vi "Sweep Control.vi"(1 "Stop":bool, 4 "Experiment Description":string="IV measurements at 0T\n- Sweep priority 0: +x gate from -10V to 10V in steps of 500mV (-x 10 to -10)\n- priority 1:+y gate from -10V to 10V in steps of 500mV (-y 10 to -10)\n- 1 IV curves at each Vsg\n- KH channel 17,18,19,20: leads 3,8,15,21\n- 5 s wait\n\nVbg = lead 26: 0V\nT: 20mK\nB=0T\n\nhash device\n\nKH channel 10,13: leads 16,27 , current mode, 5k resistor, 1000x gain\nlead 16: 3mV ac+ 1mV dc bias, 1 Hz\nKH channel 11,12: V1+/-: 17/20, 100x gain\nKH channel 5: dV: 17-20, 100x gain\n\nstripe device\n\nKH channel 7,8: leads 11,12 , current mode, 5k resistor, 1000x gain\nlead 12: 3.5mV ac+ 0mV dc bias, 1 Hz\nKH channel 6,9: V1+/-: 9,13, 100x gain\nKH channel 16: dV: 11-12, 100x gain", 5 "Experiment subVI":T9, 6 "Sweep Lockin":T1[](array[typedef]) {"Channels"."Table" format="%#_1f"; "Channels"."Channel" min=1 max=128; "Channels"."Start" format="%#_6p"; "Channels"."End" format="%#_6p"}, 7 "Experiment Folder (## - Description)":string="35-2D_0T_IV_hash_stripe", 8 "error in (no error)":errorcluster, 9 "Post action (indexing priority)":T10=[enum."Do Nothing", enum."Do Nothing", enum."Do Nothing", enum."Do Nothing"], 10 "Scan parameters":T12=[{"Start"=0.0, "End"=0.0, "Step"=0.0, "Rate"=0.0, "Waveform type"=enum."linear", "wait (ms or K)"=0.0, "Address"="Dev2/ao0", "channel"=17}, {"Start"=0.0, "End"=0.0, "Step"=0.0, "Rate"=0.0, "Waveform type"=enum."linear", "wait (ms or K)"=0.0, "Address"="Dev2/ao0", "channel"=18}, {"Start"=0.0, "End"=0.0, "Step"=0.0, "Rate"=0.0, "Waveform type"=enum."linear", "wait (ms or K)"=0.0, "Address"="Dev2/ao0", "channel"=19}, {"Start"=0.0, "End"=0.0, "Step"=0.0, "Rate"=0.0, "Waveform type"=enum."linear", "wait (ms or K)"=0.0, "Address"="Dev2/ao0", "channel"=20}] {"Rate" format="%.2f"; "Step" format="%#_6p"; "End" format="%#_6p"; "Start" format="%#_6p"}, 11 "Scan control":T14=[{"Priority"=enum."Priority 0", "Scan name"=enum."Lockin Bias"}, {"Priority"=enum."Priority 1", "Scan name"=enum."Lockin Bias"}, {"Priority"=enum."Priority 0", "Scan name"=enum."Lockin Bias"}, {"Priority"=enum."Priority 1", "Scan name"=enum."Lockin Bias"}]) -> (0 "error out":errorcluster)   [LabVIEW 2019, in "SMO.SweepControl.lvclass"]
doc: "- Priority 0 is the fastest loop\n- You can put multiple scan names in one priority.\n- OFF has to be the last priority\n- Choose an Experiment (Lockin_Sweep, IV, etc) to run at each Scan Setting\n- Open the Exeriment subVIs to choose settings"
uses:
  SMO.SweepControl.lvclass
  Typedefs/Enum - Priority.ctl
  Typedefs/Enum - Action.ctl
  Typedefs/Cluster - ScanControl.ctl
  Typedefs/ScanControl.ctl
  Typedefs/Cluster - ScanParamters.ctl
  Typedefs/ScanParamters.ctl
  Typedefs/Enum - Experiments.ctl
  Typedefs/Sweep Control JSON--Cluster.ctl
  SMO.Control Experiment/SMO.Control Experiment.lvclass
  Control Experiment SM/Control Experiment SM.lvclass
  Typedefs/Enum - PostAction.ctl
  Typedefs/PostAction.ctl
  Typedefs/Enum - PostAction - 2.ctl
  Typedefs/Cluster - Sweep Control.ctl
  <userlib>/LevyLab/Lockin-Multichannel/Instrument.DAQ/Typedefs/Sweep.Pattern--Enum.ctl
  <userlib>/LevyLab/Lockin-Multichannel/Instrument.DAQ/Instrument.DAQ.lvclass
  <userlib>/LevyLab/Lockin-Multichannel/Instrument.DAQ/Typedefs/Sweep.Channel--Cluster.ctl
  <userlib>/LevyLab/Lockin-Multichannel/Instrument.DAQ/Typedefs/Sweep.Channel--Cluster--Array.ctl
  <userlib>/LevyLab/Lockin-Multichannel/Instrument.DAQ/Typedefs/Sweep.Configuration--Cluster.ctl
panel:
  out "Repeat #":i32
  in  "Repeat Experiment":i32=1 caption="Repeat Experiment (at each parameter)" min=1
  in  "Scan parameters 2":T5[](array[typedef]) {"Rate" format="%.2f"; "Step" format="%#_6p"; "End" format="%#_6p"; "Start" format="%#_6p"}
  # "1. Scan Parameters. Choose parameters at which each experiment will take place."
  # "2. Experiment"
  # "3. If your chosen experiment is \"Lockin Sweep\", then the following sequence of sweeps will be executed at each scan parameter. (Ex. 1. Set B. 2. Set Set Vsg. 3. Lockin Sweep 1. 4. Lockin Sweep 2. Etc."
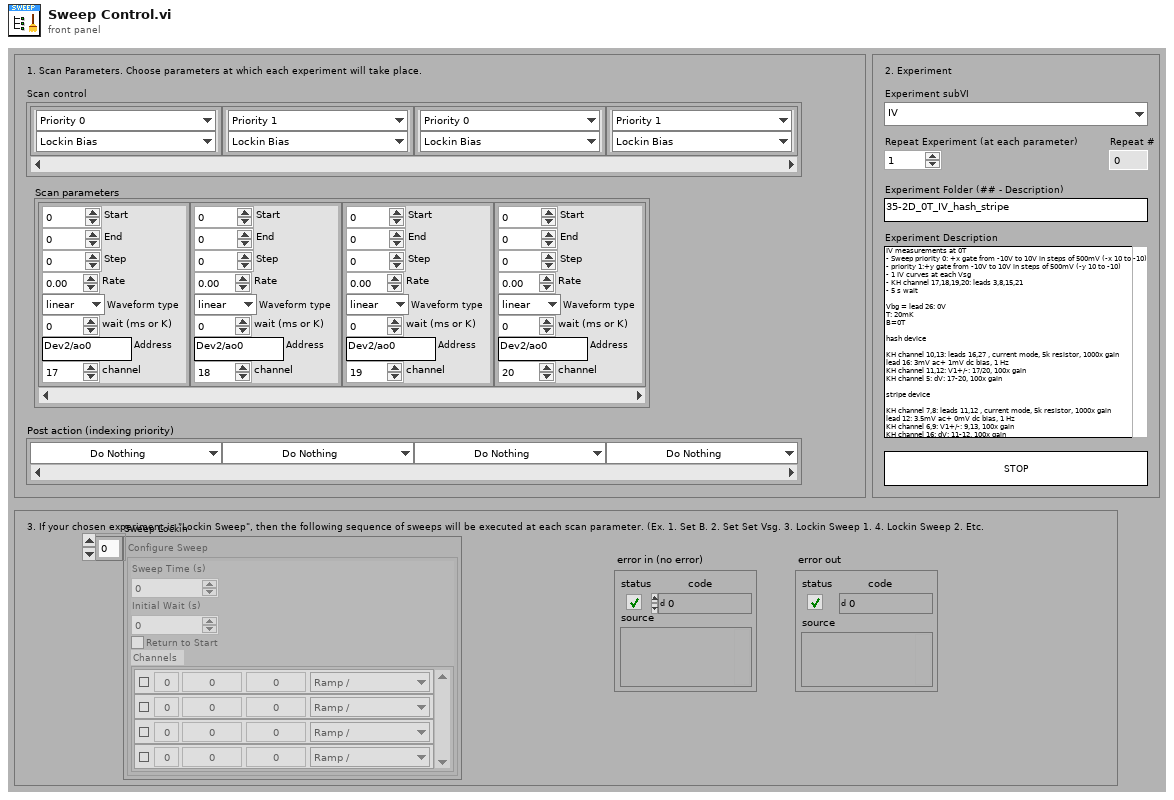
[diagram p1: front panel]
types:
  T1 = typedef "Instrument.DAQ.lvclass/Sweep.Configuration--Cluster.ctl" = cluster{"Sweep Time (s)":dbl, "Initial Wait (s)":dbl, "Return to Start":bool, "Channels":T2}
  T2 = typedef "Instrument.DAQ.lvclass/Sweep.Channel--Cluster--Array.ctl" = T3[]
  T3 = typedef "Instrument.DAQ.lvclass/Sweep.Channel--Cluster.ctl" = cluster{"Enable?":bool, "Channel":u16, "Start":dbl, "End":dbl, "Pattern":T4, "Table":dbl[]}
  T4 = typedef "Instrument.DAQ.lvclass/Sweep.Pattern--Enum.ctl" = enum16{"Ramp /", "Ramp /\\", "Smooth Ramp _/", "Smooth Ramp _/\\_", "Table"}
  T5 = typedef "SMO.SweepControl.lvclass/Cluster - Sweep Control.ctl" = cluster{"Start":dbl, "End":dbl, "Step":dbl, "Rate":dbl, "wait (ms/mK)":u32, "Address":string, "Priority":T6, "Scan name":T7, "Post Actions":T8[], "channel":i32}
  T6 = typedef "SMO.SweepControl.lvclass/Enum - Priority.ctl" = enum16{"Priority 0", "Priority 1", "Priority 2", "Priority 3", "Priority 4", "Priority 5"}
  T7 = typedef "SMO.SweepControl.lvclass/Enum - Action.ctl" = enum16{"OFF", "time", "Lockin Amplitude", "Lockin Frequency", "Lockin Bias", "Delay", "Strain", "DAQ Bias", "Magnet Field", "Temperature", "MW f1", "MW f2", "MW Amplitude1", "MW Amplitude2"}
  T8 = typedef "SMO.SweepControl.lvclass/Enum - PostAction - 2.ctl" = enum16{"Do Nothing", "Wait (time)", "Wait (Temperature)", "Wait (<T ; B sweep)", "Wait (Magnet)"}
  T9 = typedef "SMO.SweepControl.lvclass/Enum - Experiments.ctl" = enum16{"IV", "IV_Fast", "THz_DelayLine", "Lockin_Vsg", "Lockin_Sweep", "Lockin_Time", "AI WFM time", "Lockin (experimental)"}
  T10 = typedef "SMO.SweepControl.lvclass/PostAction.ctl" = T11[]
  T11 = typedef "SMO.SweepControl.lvclass/Enum - PostAction.ctl" = enum16{"Do Nothing", "Wait (time)", "Wait (Temperature)", "Wait (<T ; B sweep)", "Wait (Magnet)"}
  T12 = typedef "SMO.SweepControl.lvclass/ScanParamters.ctl" = T13[]
  T13 = typedef "SMO.SweepControl.lvclass/Cluster - ScanParamters.ctl" = cluster{"Start":dbl, "End":dbl, "Step":dbl, "Rate":dbl, "Waveform type":enum16{"linear", "triangle", "power"}, "wait (ms or K)":dbl, "Address":string, "channel":i32}
  T14 = typedef "SMO.SweepControl.lvclass/ScanControl.ctl" = T15[]
  T15 = typedef "SMO.SweepControl.lvclass/Cluster - ScanControl.ctl" = cluster{"Priority":T6, "Scan name":T7}
  T16 = enum32{"Invalid", "Standard", "Closed", "Hidden", "Minimized", "Maximized"}
  T17 = enum32{"invalid app kind", "Development System", "Run Time System", "Student Edition", "Embedded LabVIEW", "Evaluation", "Custom"}
  T18 = cluster{"Core":cluster{"Current VI Reference":refnum<vi>, "Close Panel on Exit?":bool}, "SweepControl":refnum<class "SMO.SweepControl.lvclass">}
  T19 = cluster{"Current VI Reference":refnum<vi>, "Close Panel on Exit?":bool}
  T20 = typedef "SMO.SweepControl.lvclass/Sweep Control JSON--Cluster.ctl" = cluster{"Experiment":T9, "Repeat Experiment":i32, "Scan control":T14, "Scan parameters":T12}
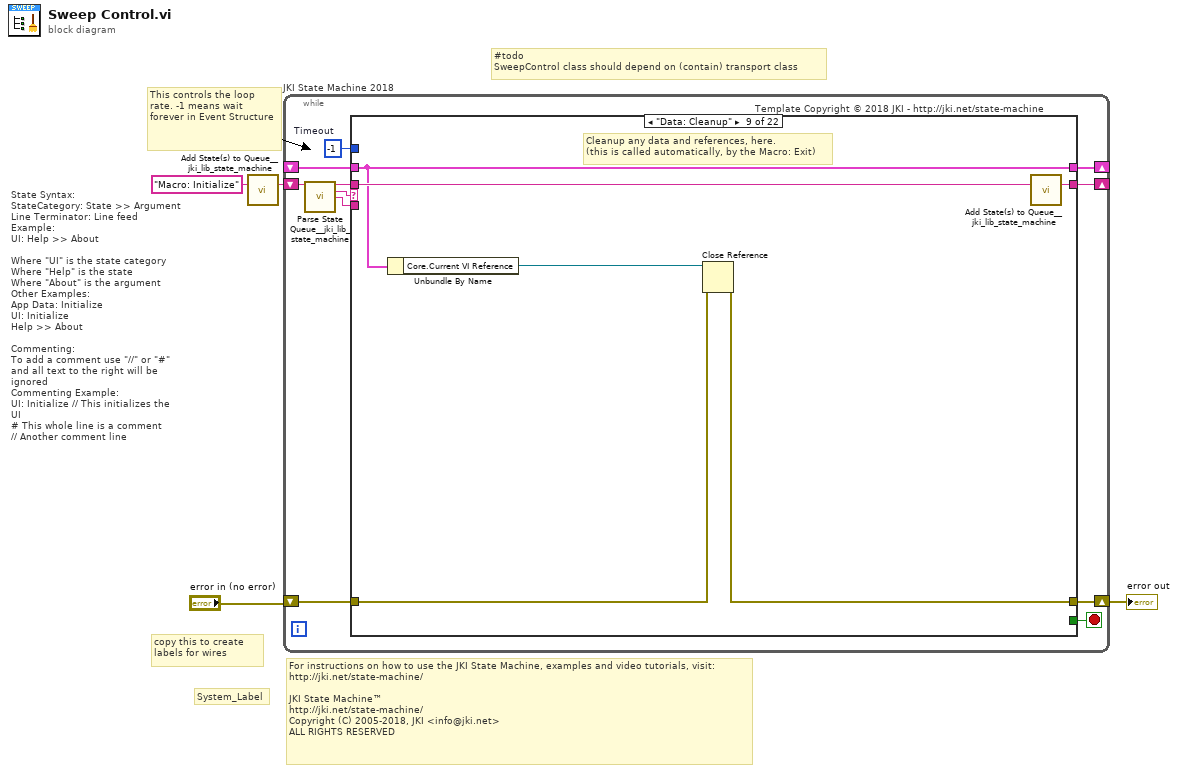
[diagram p0: block diagram]
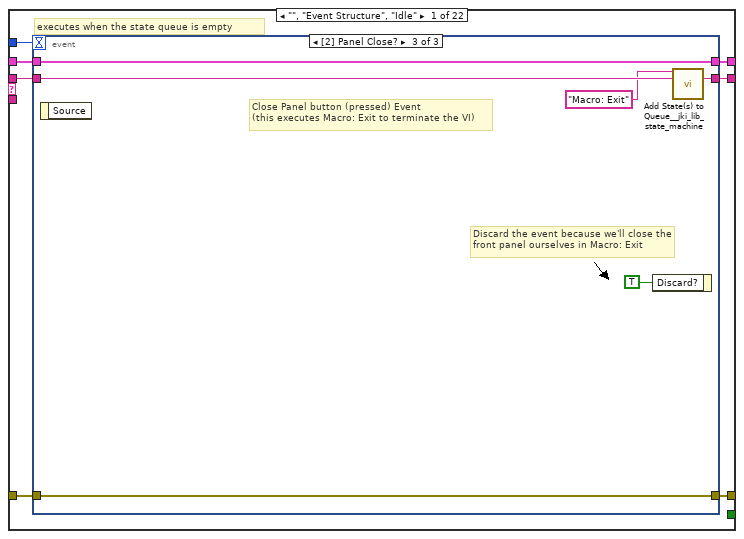
[diagram p2: hidden frame]
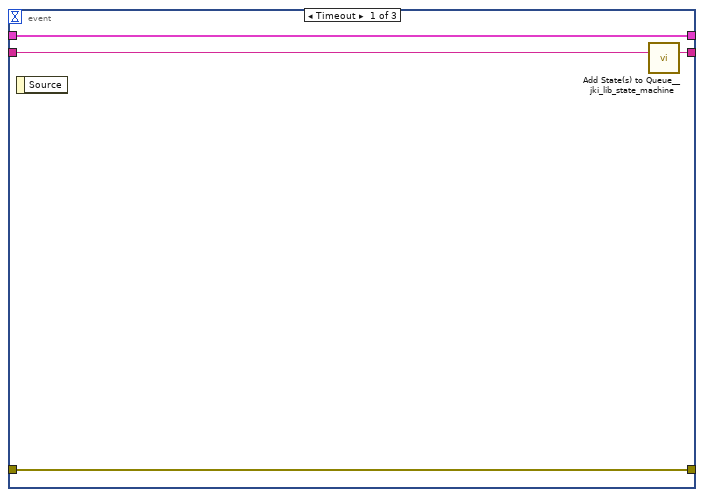
[diagram p3: hidden frame]
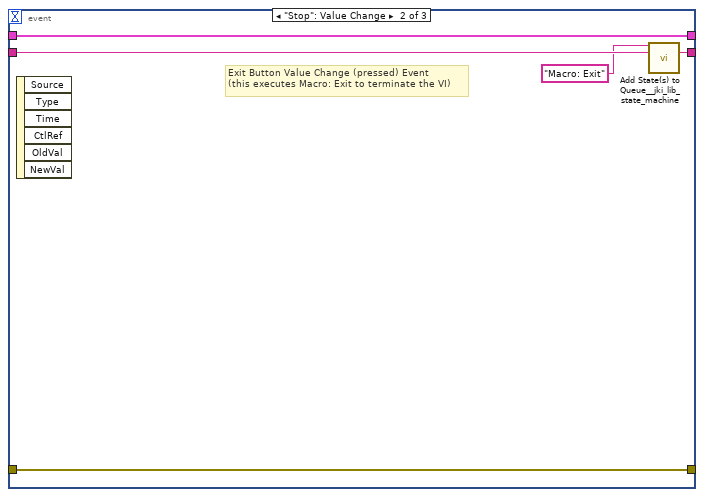
[diagram p4: hidden frame]
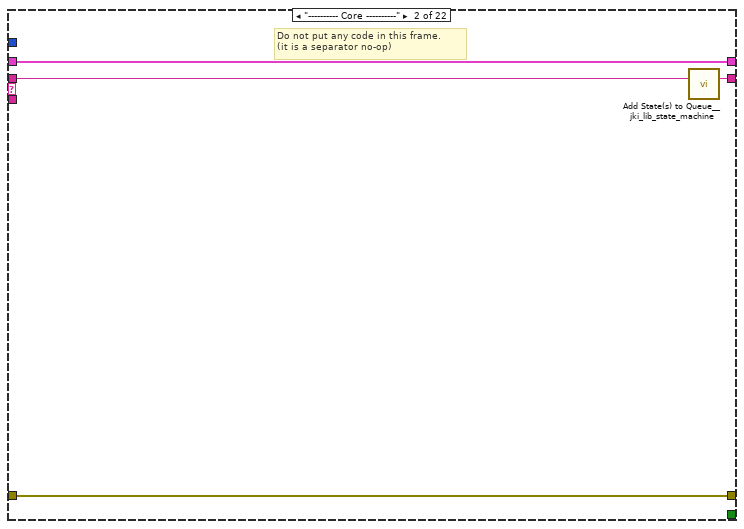
[diagram p5: hidden frame]
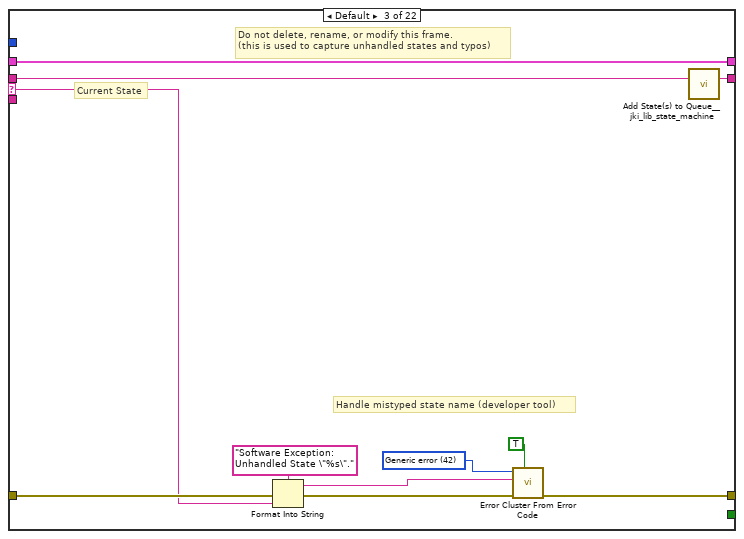
[diagram p6: hidden frame]
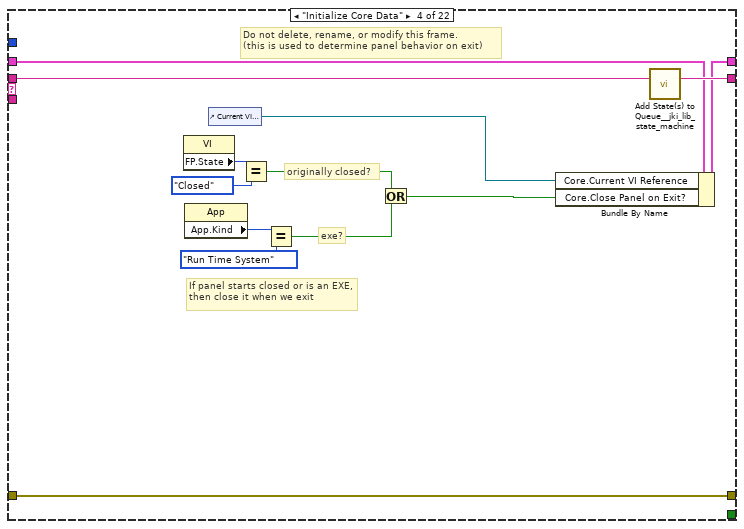
[diagram p7: hidden frame]
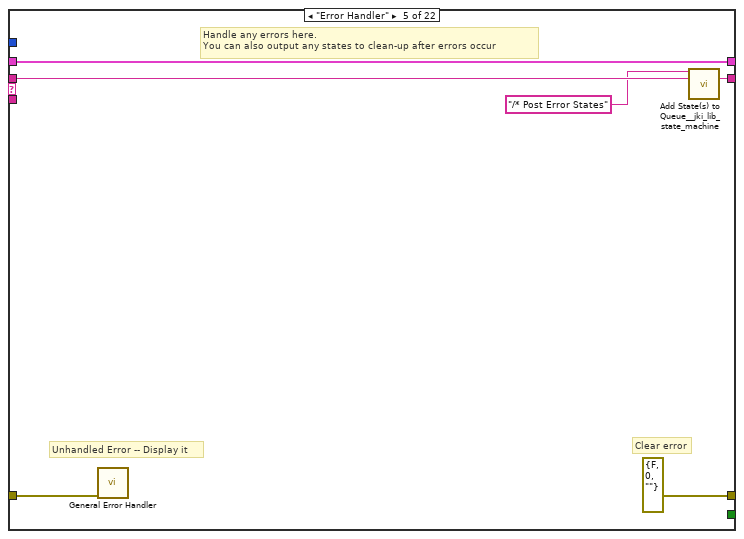
[diagram p8: hidden frame]
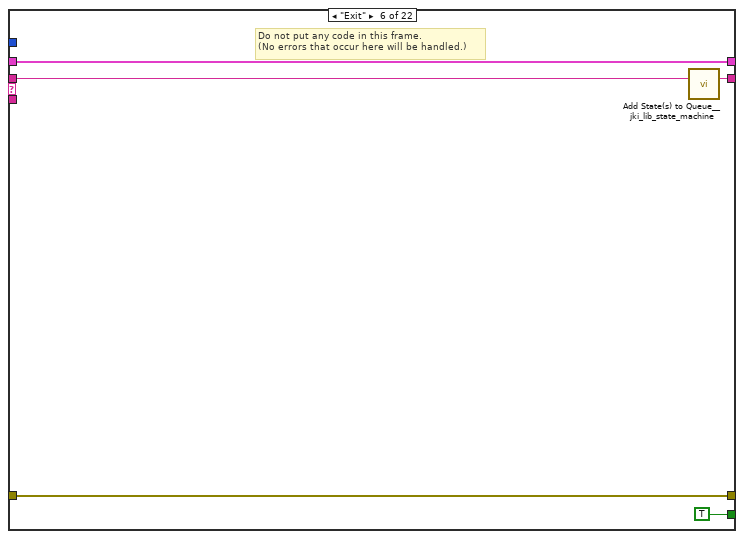
[diagram p9: hidden frame]
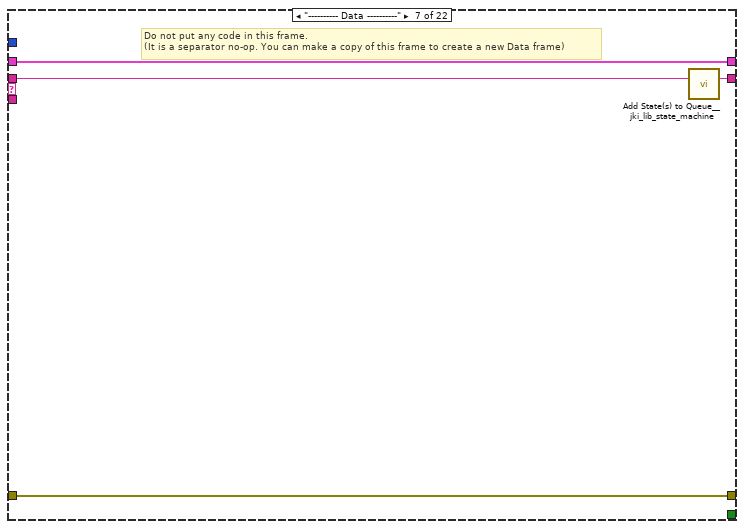
[diagram p10: hidden frame]
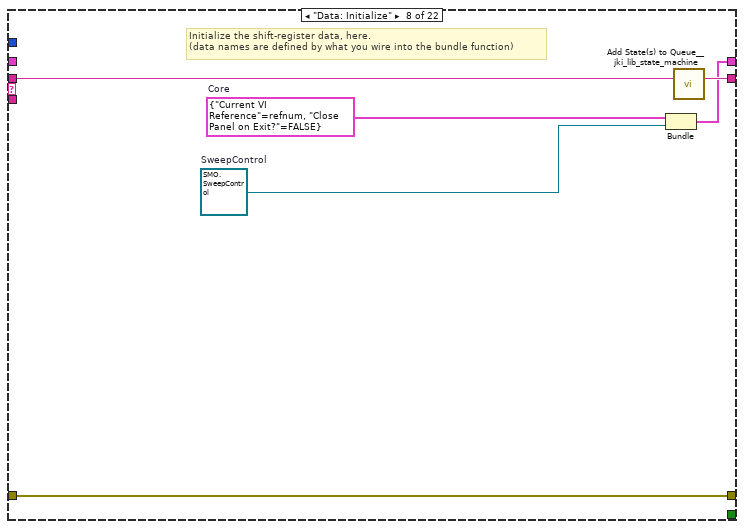
[diagram p11: hidden frame]
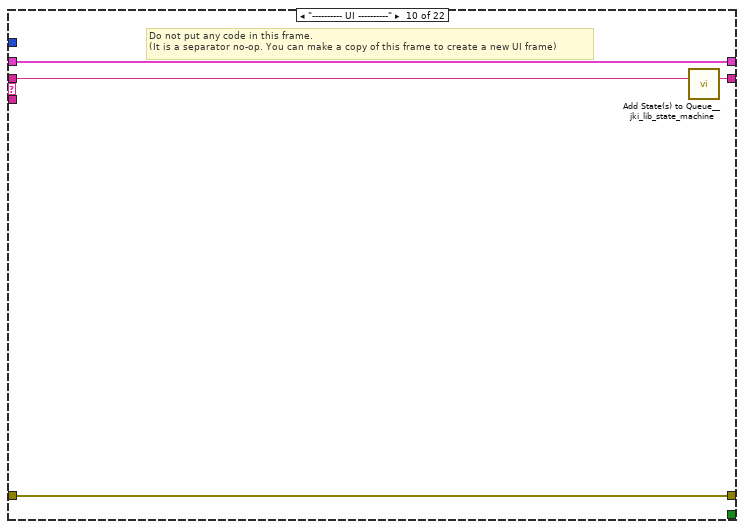
[diagram p12: hidden frame]
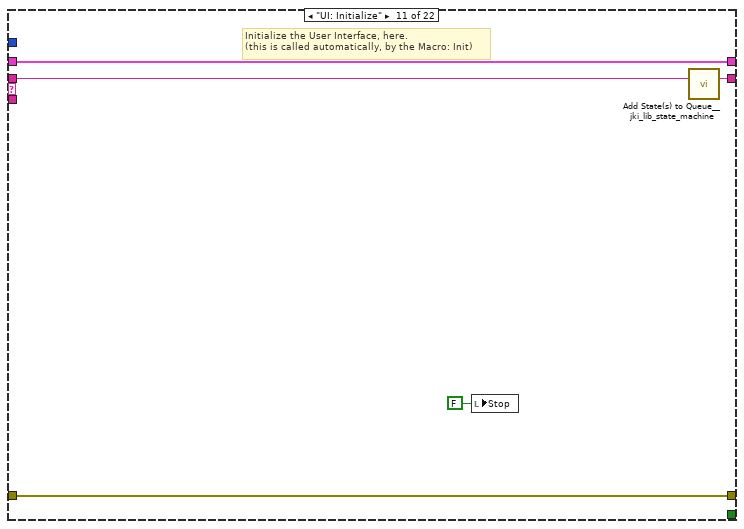
[diagram p13: hidden frame]
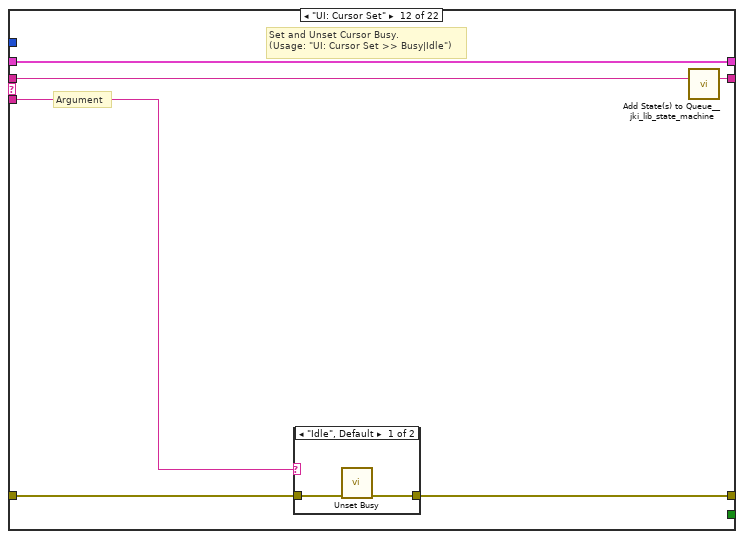
[diagram p14: hidden frame]
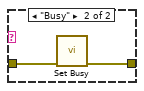
[diagram p15: hidden frame]
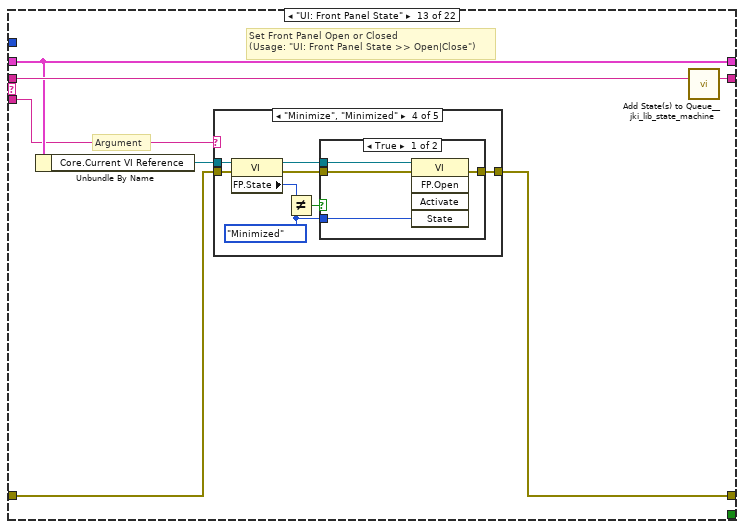
[diagram p16: hidden frame]
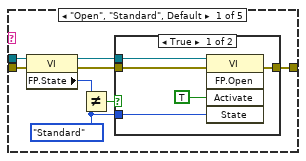
[diagram p17: hidden frame]
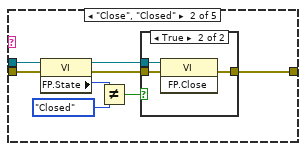
[diagram p19: hidden frame]
diagram:
  # "For instructions on how to use the JKI State Machine, examples and video tutorials, visit:\nhttp://jki.net/state-machine/\n\nJKI State Machine™\nhttp://jki.net/state-machine/\nCopyright (C) 2005-2018, JKI <info@jki.net>\nALL RIGHTS RESERVED"
  # "State Syntax:\nStateCategory: State >> Argument\nLine Terminator: Line feed\nExample:\nUI: Help >> About\n\nWhere \"UI\" is the state category\nWhere \"Help\" is the state\nWhere \"About\" is the argument\nOther Examples:\nApp Data: Initialize\nUI: Initialize\nHelp >> About\n\nCommenting:\nTo add a comment use \"//\" or \"#\" and all text to the right will be ignored\nCommenting Example:\nUI: Initialize // This initializes the UI\n# This whole line is a comment\n// Another comment line"
  # "copy this to create labels for wires"
  # "This controls the loop rate. -1 means wait forever in Event Structure"
  # "System_Label"
  # "#todo\nSweepControl class should depend on (contain) transport class"
  n1 = call <vilib>:"Add State(s) to Queue__jki_lib_state_machine.vi"("State(s) in (\"\")"="Macro: Initialize") -> ("States Out"=w4:string)  [unwired: 14 in]
  n2 = while "JKI State Machine 2018" {
    shift-right: [w8] -> _
    shift-left: _ -> [w7]
    shift-right: [w11] -> w1
    shift-left: "error in (no error)" -> [w5]
    shift-right: [w10] -> _
    shift-left: w4 -> [w12]
    stop <- w9 stop-if-true
    w6 = -1  # Timeout
    # "Template Copyright © 2018 JKI - http://jki.net/state-machine"
    n3 = call <vilib>:"Parse State Queue__jki_lib_state_machine.vi"("State Queue"=w12) -> ("Remaining States"=w14:string, "Current State"=w15:string, "Arguments"=w13:string)  [unwired: 12 in]
    n4 = case shown="\"Data: Cleanup\"" w15 {
      selector: w15 -> [_ _ w42 _ _ _ _ _ _ _ _ _ _ _ _ _ _ _ _ _ _ _]
      tunnel: w14 -> [w22 w41 w46 w65 w71 w76 w80 w86 w92 w96 w101 w107 w118 w187 w192 w197 w208 w212 w238 w251 w256 w264]
      tunnel: w13 -> [_ _ _ _ _ _ _ _ _ _ _ w102 w112 _ _ _ _ _ _ _ _ _]
      tunnel: w7 -> [w20 w38 w44 w58 w68 w74 w77 _ w87 w93 w99 w105 w114 w184 w189 w194 w205 w209 w232 w249 w254 w260]
      tunnel: [w19 w39 w48 w62 errorcluster {"status"=FALSE, "code"=0, "source"=""} ("error out") w73 w78 w83 w88 w94 w98 w103 w115 w185 w190 w195 w206 w210 w230 w247 w252 w263] -> w11
      tunnel: w5 -> [w18 w39 w47 w62 w67 w73 w78 w83 w89 w94 w98 w104 w116 w185 w190 w195 w206 w210 w226 w239 w252 w263]
      tunnel: [w21 w40 w45 w64 w70 w75 w79 w85 w91 w95 w100 w106 w117 w186 w191 w196 w207 w211 w237 w250 w255 w265] -> w10
      tunnel: [_ _ _ _ _ TRUE _ _ _ _ _ _ _ _ _ _ _ _ _ _ _ _] -> w9
      tunnel: [w17 w38 w44 w63 w68 w74 w77 w84 w87 w93 w99 w105 w114 w184 w189 w194 w205 w209 w231 w249 w254 w259] -> w8
      tunnel: w6 -> [w16 _ _ _ _ _ _ _ _ _ _ _ _ _ _ _ _ _ _ _ _ _]
      frame "", "Event Structure", "Idle" {
        # "executes when the state queue is empty"
        n5 = event shown="[2] Panel Close?" {
          selector: _ -> [_ _ _]
          dyn-events: _ -> [_ _ _]
          timeout: w16 -> [_ _ _]
          tunnel: w22 -> [w26 w31 w37]
          tunnel: [w25 w30 w36] -> w21
          tunnel: w20 -> [w23 w28 w34]
          tunnel: [w24 w29 w35] -> w19
          tunnel: w18 -> [w24 w29 w35]
          tunnel: [w23 w28 w34] -> w17
          event Timeout {
            n6 = event-data() -> ()  [unwired: 1 in, 1 out]
            n7 = call <vilib>:"Add State(s) to Queue__jki_lib_state_machine.vi"("State(s) in (\"\")"=w26) -> ("States Out"=w25:string)  [unwired: 14 in]
          }
          event "Stop": Value Change {
            # "Exit Button Value Change (pressed) Event\n(this executes Macro: Exit to terminate the VI)"
            n8 = event-data() -> ()  [unwired: 1 in, 6 out]
            n9 = call <vilib>:"Add State(s) to Queue__jki_lib_state_machine.vi"("State(s) in Front (\"\")"="Macro: Exit", "State(s) in (\"\")"=w31) -> ("States Out"=w30:string)  [unwired: 13 in]
          }
          event Panel Close? {
            # "Discard the event because we'll close the front panel ourselves in Macro: Exit"
            # "Close Panel button (pressed) Event\n(this executes Macro: Exit to terminate the VI)"
            n10 = event-data() -> ()  [unwired: 1 in, 1 out]
            n11 = event-data("Discard?"=TRUE) -> ()  [unwired: 1 in, 1 out]
            n12 = call <vilib>:"Add State(s) to Queue__jki_lib_state_machine.vi"("State(s) in Front (\"\")"="Macro: Exit", "State(s) in (\"\")"=w37) -> ("States Out"=w36:string)  [unwired: 13 in]
          }
        }
      }
      frame "---------- Core ----------" {
        # "Do not put any code in this frame.\n(it is a separator no-op)"
        n13 = call <vilib>:"Add State(s) to Queue__jki_lib_state_machine.vi"("State(s) in (\"\")"=w41) -> ("States Out"=w40:string)  [unwired: 14 in]
      }
      frame Default {
        w51 = 42 items=["No error", "Argument error", "Memory is full", "Out of zone", "End of file", "File already open", "Generic file I/O error", "File not found", "File permission error", "Disk is full", "Duplicate path", "Too many files open", "System feature not enabled", "Resource file not found", "Cannot add resource", "Resource not found", "Image not found", "Image memory error", "Pen does not exist", "Config type invalid", "Config token not found", "Config parse error", "Config memory error", "Bad external code format", "Bad external code offset", "External code not present", "Null window", "Destroy window error", "Null menu", "Print aborted", "Bad print record", "Print driver error", "Windows error during printing", "Memory error during printing", "Print dialog error", "Generic print error", "Invalid device refnum", "Device not found", "Device parameter error", "Device unit error", "Cannot open device", "Device call aborted", "Generic error", "Cancelled by user", "Object ID too low", "Object ID too high", "Object not in heap", "Unknown heap", "Unknown object (invalid DefProc)", "Unknown object (DefProc not in table)", "Message out of range", "Invalid (null) method", "Unknown message", "Manager call not supported", "Bad address", "Network operation in progress", "Network operation timed out", "Connection is busy", "Network attribute not supported", "Network error", "Address in use", "System out of memory", "Connection aborted", "Connection refused", "Not connected", "Already connected", "Connection closed", "Initialization error (interapplication manager)", "Bad occurrence", "Wait on unbound occurrence handler", "Occurrence queue overflow", "Datalog type conflict", "Unused", "Unrecognized type (interapplication manager)", "Memory corrupt", "Failed to make temporary DLL", "Old CIN version", "Drag socket not found", "Failed to load drop-object", "Failed to register OLE object", "Failed to release OLE object", "Format specifier type mismatch", "Unknown format specifier", "Too few format specifiers", "Too many format specifiers", "Scan failed", "Newer CIN version", "Error converting to variant", "Runtime menu error", "Password tampered", "Variant attribute not found", "Incompatible variant data type", "Event data is not available", "Event Store is not present", "Occurrence is not found", "Event Queue is not created", "Event info is not available", "Refnum passed is NULL", "Error retrieving Class GUID", "Error retrieving CoClass GUID", "Error retrieving TypeLib GUID.", "Bad built application magic bytes.", "Specific driver is different from the specific driver associated with the Logical Name.", "There is no session opened to the class driver.", "Max Error", "MAX - Error with config objects", "MAX - Error loading configuration", "MAX - Group not supported"]
        # "Current State"
        # "Do not delete, rename, or modify this frame.\n(this is used to capture unhandled states and typos)"
        # "Handle mistyped state name (developer tool)"
        n14 = Format Into String(format string="Software Exception: Unhandled State \"%s\"." ("message"), error in=w47, w42) -> (resulting string=w50:string, error out=w49:errorcluster)  [unwired: 1 in]
        n15 = call <vilib>:"Error Cluster From Error Code.vi"("show call chain? (False)"=TRUE, "error in (no error)"=w49, "error message (\"\")"=w50, "error code (0)"=w51) -> ("error out"=w48:errorcluster)  [unwired: 5 in]
        n16 = call <vilib>:"Add State(s) to Queue__jki_lib_state_machine.vi"("State(s) in (\"\")"=w46) -> ("States Out"=w45:string)  [unwired: 14 in]
      }
      frame "Initialize Core Data" {
        # "Do not delete, rename, or modify this frame.\n(this is used to determine panel behavior on exit)"
        # "originally closed?"
        # "exe?"
        # "If panel starts closed or is an EXE, then close it when we exit"
        n17 = property class="VI"() -> ("FP.State"=w55:T16)  [unwired: 2 in, 2 out]
        n18 = property class="App"() -> ("App.Kind"=w61:T17)  [unwired: 2 in, 2 out]
        n19 = control-ref of="Current VI Reference"() -> (w56:refnum<vi>)
        n20 = Equal?(x=w55, y=T16."Closed" ("Front Panel Window:State")) -> (x = y?=w53:bool)
        n21 = Equal?(x=w61, y=T17."Run Time System" ("Application:Kind")) -> (x = y?=w59:bool)
        n22 = Or(x=w53, y=w59) -> (x .or. y?=w57:bool)
        n23 = Bundle By Name(cluster=w58, "Core.Current VI Reference"=w56, "Core.Close Panel on Exit?"=w57) -> (w63:T18)
        n24 = call <vilib>:"Add State(s) to Queue__jki_lib_state_machine.vi"("State(s) in (\"\")"=w65) -> ("States Out"=w64:string)  [unwired: 14 in]
      }
      frame "Error Handler" {
        # "Unhandled Error -- Display it"
        # "Handle any errors here.\nYou can also output any states to clean-up after errors occur"
        # "Clear error"
        n25 = call <vilib>:"General Error Handler.vi"("error in (no error)"=w67) -> ()  [unwired: 10 in, 5 out]
        n26 = call <vilib>:"Add State(s) to Queue__jki_lib_state_machine.vi"("State(s) in Front (\"\")"="/* Post Error States", "State(s) in (\"\")"=w71) -> ("States Out"=w70:string)  [unwired: 13 in]
      }
      frame "Exit" {
        # "Do not put any code in this frame.\n(No errors that occur here will be handled.)"
        n27 = call <vilib>:"Add State(s) to Queue__jki_lib_state_machine.vi"("State(s) in (\"\")"=w76) -> ("States Out"=w75:string)  [unwired: 14 in]
      }
      frame "---------- Data ----------" {
        # "Do not put any code in this frame.\n(It is a separator no-op. You can make a copy of this frame to create a new Data frame)"
        n28 = call <vilib>:"Add State(s) to Queue__jki_lib_state_machine.vi"("State(s) in (\"\")"=w80) -> ("States Out"=w79:string)  [unwired: 14 in]
      }
      frame "Data: Initialize" {
        w81 = refnum<class "SMO.SweepControl.lvclass"> refnum  # SweepControl
        w82 = T19 {"Current VI Reference"=refnum, "Close Panel on Exit?"=FALSE}  # Core
        # "Initialize the shift-register data, here.\n(data names are defined by what you wire into the bundle function)"
        n29 = Bundle("Core"=w82, "SweepControl"=w81) -> (w84:T18)  [unwired: 1 in]
        n30 = call <vilib>:"Add State(s) to Queue__jki_lib_state_machine.vi"("State(s) in (\"\")"=w86) -> ("States Out"=w85:string)  [unwired: 14 in]
      }
      frame "Data: Cleanup" {
        # "Cleanup any data and references, here.\n(this is called automatically, by the Macro: Exit)"
        n31 = Unbundle By Name(w87) -> ("Core.Current VI Reference"=w90:refnum<vi>)
        n32 = Close Reference(reference=w90, error in (no error)=w89) -> (error out=w88:errorcluster)
        n33 = call <vilib>:"Add State(s) to Queue__jki_lib_state_machine.vi"("State(s) in (\"\")"=w92) -> ("States Out"=w91:string)  [unwired: 14 in]
      }
      frame "---------- UI ----------" {
        # "Do not put any code in this frame.\n(It is a separator no-op. You can make a copy of this frame to create a new UI frame)"
        n34 = call <vilib>:"Add State(s) to Queue__jki_lib_state_machine.vi"("State(s) in (\"\")"=w96) -> ("States Out"=w95:string)  [unwired: 14 in]
      }
      frame "UI: Initialize" {
        # "Initialize the User Interface, here.\n(this is called automatically, by the Macro: Init)"
        n35 = local write "Stop"(FALSE ("Stop")) -> ()
        n36 = call <vilib>:"Add State(s) to Queue__jki_lib_state_machine.vi"("State(s) in (\"\")"=w101) -> ("States Out"=w100:string)  [unwired: 14 in]
      }
      frame "UI: Cursor Set" {
        # "Argument"
        # "Set and Unset Cursor Busy.\n(Usage: \"UI: Cursor Set >> Busy|Idle\")"
        n37 = case shown="\"Idle\", Default" w102 {
          tunnel: w104 -> [w109 w111]
          tunnel: [w108 w110] -> w103
          frame "Idle", Default {
            n38 = call <vilib>:"Unset Busy.vi"("error in (no error)"=w109) -> ("error out"=w108:errorcluster)  [unwired: 10 in]
          }
          frame "Busy" {
            n39 = call <vilib>:"Set Busy.vi"("error in (no error)"=w111) -> ("error out"=w110:errorcluster)  [unwired: 9 in, 1 out]
          }
        }
        n40 = call <vilib>:"Add State(s) to Queue__jki_lib_state_machine.vi"("State(s) in (\"\")"=w107) -> ("States Out"=w106:string)  [unwired: 14 in]
      }
      frame "UI: Front Panel State" {
        # "Argument"
        # "Set Front Panel Open or Closed\n(Usage: \"UI: Front Panel State >> Open|Close\")"
        n41 = Unbundle By Name(w114) -> ("Core.Current VI Reference"=w113:refnum<vi>)
        n42 = case shown="\"Minimize\", \"Minimized\"" w112 {
          tunnel: w116 -> [w124 w139 w150 w163 w176]
          tunnel: [w126 w140 w152 w165 w178] -> w115
          tunnel: w113 -> [w125 w137 w151 w164 w177]
          frame "Open", "Standard", Default {
            w119 = T16."Standard" ("State")
            n43 = property class="VI"(reference=w125, error in=w124) -> (reference out=w122:refnum<vi>, error out=w123:errorcluster, "FP.State"=w121:T16)
            n44 = Not Equal?(x=w121, y=w119) -> (x != y?=w120:bool)
            n45 = case shown="True" w120 {
              tunnel: [w130 w132] -> w126
              tunnel: w123 -> [w129 w132]
              tunnel: w122 -> [w128 _]
              tunnel: w119 -> [w127 _]
              frame True {
                n46 = invoke class="VI" method="FP.Open"(reference=w128, error in=w129, "Activate"=TRUE, "State"=w127) -> (error out=w130:errorcluster)  [unwired: 1 in, 4 out]
              }
              frame False {
              }
            }
          }
          frame "Close", "Closed" {
            n47 = property class="VI"(reference=w137, error in=w139) -> (reference out=w136:refnum<vi>, error out=w138:errorcluster, "FP.State"=w134:T16)
            n48 = Not Equal?(x=w134, y=T16."Closed" ("Front Panel Window:State")) -> (x != y?=w133:bool)
            n49 = case shown="True" w133 {
              tunnel: [w141 w144] -> w140
              tunnel: w138 -> [w141 w143]
              tunnel: w136 -> [_ w142]
              frame False {
              }
              frame True {
                n50 = invoke class="VI" method="FP.Close"(reference=w142, error in=w143) -> (error out=w144:errorcluster)  [unwired: 1 in, 2 out]
              }
            }
          }
          frame "Hidden", "Hide" {
            w145 = T16."Hidden" ("State")
            n51 = property class="VI"(reference=w151, error in=w150) -> (reference out=w148:refnum<vi>, error out=w149:errorcluster, "FP.State"=w147:T16)
            n52 = Not Equal?(x=w147, y=w145) -> (x != y?=w146:bool)
            n53 = case shown="True" w146 {
              tunnel: [w156 w157] -> w152
              tunnel: w149 -> [w155 w157]
              tunnel: w148 -> [w154 _]
              tunnel: w145 -> [w153 _]
              frame True {
                n54 = invoke class="VI" method="FP.Open"(reference=w154, error in=w155, "State"=w153) -> (error out=w156:errorcluster)  [unwired: 2 in, 4 out]
              }
              frame False {
              }
            }
          }
          frame "Minimize", "Minimized" {
            w158 = T16."Minimized" ("State")
            n55 = property class="VI"(reference=w164, error in=w163) -> (reference out=w161:refnum<vi>, error out=w162:errorcluster, "FP.State"=w160:T16)
            n56 = Not Equal?(x=w160, y=w158) -> (x != y?=w159:bool)
            n57 = case shown="True" w159 {
              tunnel: [w169 w170] -> w165
              tunnel: w162 -> [w168 w170]
              tunnel: w161 -> [w167 _]
              tunnel: w158 -> [w166 _]
              frame True {
                n58 = invoke class="VI" method="FP.Open"(reference=w167, error in=w168, "State"=w166) -> (error out=w169:errorcluster)  [unwired: 2 in, 4 out]
              }
              frame False {
              }
            }
          }
          frame "Maximize", "Maximized" {
            w171 = T16."Maximized" ("State")
            n59 = property class="VI"(reference=w177, error in=w176) -> (reference out=w174:refnum<vi>, error out=w175:errorcluster, "FP.State"=w173:T16)
            n60 = Not Equal?(x=w173, y=w171) -> (x != y?=w172:bool)
            n61 = case shown="True" w172 {
              tunnel: [w182 w183] -> w178
              tunnel: w175 -> [w181 w183]
              tunnel: w174 -> [w180 _]
              tunnel: w171 -> [w179 _]
              frame True {
                n62 = invoke class="VI" method="FP.Open"(reference=w180, error in=w181, "State"=w179) -> (error out=w182:errorcluster)  [unwired: 2 in, 4 out]
              }
              frame False {
              }
            }
          }
        }
        n63 = call <vilib>:"Add State(s) to Queue__jki_lib_state_machine.vi"("State(s) in (\"\")"=w118) -> ("States Out"=w117:string)  [unwired: 14 in]
      }
      frame "---------- Macro ----------" {
        # "Do not put any code in this frame.\n(It is a separator no-op. You can make a copy of this frame to create a new Macro frame)"
        n64 = call <vilib>:"Add State(s) to Queue__jki_lib_state_machine.vi"("State(s) in (\"\")"=w187) -> ("States Out"=w186:string)  [unwired: 14 in]
      }
      frame "Macro: Initialize" {
        w188 = "Data: Initialize\nInitialize Core Data\nUI: Initialize\nUI: Front Panel State >> Open\nMacro: Sweep"  # Data: Initialize Initialize Core Data UI: Initialize UI: Front Panel State >> Open Macro: Sweep
        # "Initialization Macro\n(This is called once, when the VI starts)"
        n65 = call <vilib>:"Add State(s) to Queue__jki_lib_state_machine.vi"("State(s) in Front (\"\")"=w188, "State(s) in (\"\")"=w192) -> ("States Out"=w191:string)  [unwired: 13 in]
      }
      frame "Macro: Sweep" {
        # "Do not put any code in this frame.\n(It is a separator no-op. You can make a copy of this frame to create a new Macro frame)"
        n66 = call <vilib>:"Add State(s) to Queue__jki_lib_state_machine.vi"("State(s) in Front (\"\")"="Sweep: Initialize\nSweep: Write JSON File\nSweep: Sweep\nMacro: Exit", "State(s) in (\"\")"=w197) -> ("States Out"=w196:string)  [unwired: 13 in]
      }
      frame "Macro: Exit" {
        # "Exit Macro\n(This is called once, when the VI exits)"
        n67 = Unbundle By Name(w205) -> ("Core.Close Panel on Exit?"=w204:bool)
        n68 = Select(t="UI: Front Panel State >> Close", s=w204, f="") -> (s? t:f=w201:string)
        n69 = call <vilib>:"Add State(s) to Queue__jki_lib_state_machine.vi"("State(s) in Front (\"\")"="Sweep: Upload to AWS", "State(s) in (\"\")"=w201, "State(s) at Back (\"\")"="Data: Cleanup\nExit") -> ("States Out"=w199:string)  [unwired: 12 in]
        n70 = call <vilib>:"Add State(s) to Queue__jki_lib_state_machine.vi"("State(s) in Front (\"\")"=w199, "State(s) in (\"\")"=w208) -> ("States Out"=w207:string)  [unwired: 13 in]
      }
      frame "---------- Sweep ----------" {
        # "Template Separator\n(You can make a copy of, or modify, this frame)"
        n71 = call <vilib>:"Add State(s) to Queue__jki_lib_state_machine.vi"("State(s) in (\"\")"=w212) -> ("States Out"=w211:string)  [unwired: 14 in]
      }
      frame "Sweep: Initialize" {
        # "hidden: 1/7/2020"
        # "Your code here.\n(You can make a copy of, or modify, this frame)"
        n72 = Unbundle By Name(w232) -> ("SweepControl"=w229:refnum<class "SMO.SweepControl.lvclass">)
        n73 = call "Control Experiment FGV.vi"("Function"=enum16{"read", "write"}."read", "error in (no error)"=w226) -> ("error out"=w218:errorcluster, "Control Experiment out"=w220:refnum<class "SMO.Control Experiment.lvclass">)  [unwired: 8 in]
        n74 = call "Write Experiment Description.vi"("error in (no error)"=w218, "Experiment Description"="Experiment Description", "Control Experiment"=w220) -> ("error out"=w217:errorcluster, "Control Experiment out"=w216:refnum<class "SMO.Control Experiment.lvclass">)  [unwired: 7 in]
        n75 = call "Write Experiment Folder.vi"("error in (no error)"=w217, "Experiment Folder"="Experiment Folder (## - Description)", "Control Experiment"=w216) -> ("error out"=w222:errorcluster, "Control Experiment out"=w223:refnum<class "SMO.Control Experiment.lvclass">)  [unwired: 7 in]
        n76 = call "Read Instruments.vi"("error in (no error)"=w222, "Control Experiment"=w223) -> ("error out"=w221:errorcluster, "Control Experiment out"=w215:refnum<class "SMO.Control Experiment.lvclass">)  [unwired: 7 in, 1 out]
        n77 = Bundle By Name(cluster=w229, "Scan control"="Scan control", "Scan parameters"="Scan parameters", "Post action (indexing priority)"="Post action (indexing priority)", "Experiment"="Experiment subVI", "Control Experiment"=w215, "Scan parameters 2"="Scan parameters 2", "Sweep Lockin"="Sweep Lockin") -> (w228:refnum<class "SMO.SweepControl.lvclass">)
        n78 = call "Sort Scan Parameters.vi"("error in (no error)"=w221, "SweepControl"=w228) -> ("error out"=w230:errorcluster, "SweepControl"=w224:refnum<class "SMO.SweepControl.lvclass">)  [unwired: 6 in, 2 out]
        n79 = Bundle By Name(cluster=w232, "SweepControl"=w224) -> (w231:T18)
        n80 = call <vilib>:"Add State(s) to Queue__jki_lib_state_machine.vi"("State(s) in (\"\")"=w238) -> ("States Out"=w237:string)  [unwired: 14 in]
      }
      frame "Sweep: Write JSON File" {
        w248 = T20 {"Experiment"=enum."IV", "Repeat Experiment"=0, "Scan control"=[], "Scan parameters"=[]}  # SweepControl
        # "Write JSON File\n(Writes Sweep Control configuration to *.json file)"
        n81 = Unbundle By Name(w249) -> ("SweepControl"=w242:refnum<class "SMO.SweepControl.lvclass">)
        n82 = Unbundle By Name(w242) -> ("Control Experiment"=w241:refnum<class "SMO.Control Experiment.lvclass">)
        n83 = local read "Repeat Experiment"() -> (w240:i32)
        n84 = Unbundle By Name(w242) -> ("Scan control"=w246:T14, "Scan parameters"=w245:T12, "Experiment"=w244:T9)
        n85 = Bundle By Name(cluster=w248, "Scan control"=w246, "Scan parameters"=w245, "Experiment"=w244, "Repeat Experiment"=w240) -> (w243:T20)
        n86 = call "Save JSON File.vi"("error in (no error)"=w239, "Data"=w243, "Control Experiment"=w241) -> ("error out"=w247:errorcluster)  [unwired: 6 in, 2 out]
        n87 = call <vilib>:"Add State(s) to Queue__jki_lib_state_machine.vi"("State(s) in (\"\")"=w251) -> ("States Out"=w250:string)  [unwired: 14 in]
      }
      frame "Sweep: Upload to AWS" {
        # "Template Separator\n(You can make a copy of, or modify, this frame)"
        n88 = Unbundle By Name(w254) -> ("SweepControl"=w253:refnum<class "SMO.SweepControl.lvclass">)
        n89 = Unbundle By Name(w253) -> ()  [unwired: 1 out]
        n90 = call <vilib>:"Add State(s) to Queue__jki_lib_state_machine.vi"("State(s) in (\"\")"=w256) -> ("States Out"=w255:string)  [unwired: 14 in]
      }
      frame "Sweep: Sweep" {
        # "Your code here.\n(You can make a copy of, or modify, this frame)"
        n91 = Unbundle By Name(w260) -> ("SweepControl"=w262:refnum<class "SMO.SweepControl.lvclass">)
        n92 = while {
          tunnel: w263 -> [w275]
          tunnel: w262 -> [w277]
          tunnel: [w268] -> w258
          tunnel: [w267] -> _
          tunnel: [w266] -> w257
          i -> [w272]
          stop <- w269 stop-if-true
          w273 = 3  # loop #
          n93 = local read "Stop"() -> (w271:bool)
          n94 = call "Sweep Control Inner Loop.vi"("error in (no error)"=w275, "inner loop index"=w272, "loop #"=w273, "SweepControl in"=w277) -> ("error out"=w274:errorcluster, "Stop?"=w270:bool, "SweepControl out"=w276:refnum<class "SMO.SweepControl.lvclass">)  [unwired: 5 in]
          n95 = Or(x=w270, y=w271) -> (x .or. y?=w269:bool)
          n96 = while {
            tunnel: w274 -> [w288]
            tunnel: w276 -> [w289]
            tunnel: [w280] -> w268
            tunnel: [w279] -> w267
            tunnel: [w278] -> w266
            i -> [w284]
            stop <- w281 stop-if-true
            w287 = 2  # loop #
            n97 = local read "Stop"() -> (w283:bool)
            n98 = call "Sweep Control Inner Loop.vi"("error in (no error)"=w288, "inner loop index"=w284, "loop #"=w287, "SweepControl in"=w289) -> ("error out"=w286:errorcluster, "Stop?"=w282:bool, "SweepControl out"=w285:refnum<class "SMO.SweepControl.lvclass">)  [unwired: 5 in]
            n99 = Or(x=w282, y=w283) -> (x .or. y?=w281:bool)
            n100 = while {
              tunnel: w286 -> [w301]
              tunnel: w285 -> [w300]
              tunnel: [w292] -> w280
              tunnel: [w291] -> w279
              tunnel: [w290] -> w278
              i -> [w296]
              stop <- w293 stop-if-true
              w299 = 1  # loop #
              n101 = local read "Stop"() -> (w295:bool)
              n102 = call "Sweep Control Inner Loop.vi"("error in (no error)"=w301, "inner loop index"=w296, "loop #"=w299, "SweepControl in"=w300) -> ("error out"=w298:errorcluster, "Stop?"=w294:bool, "SweepControl out"=w297:refnum<class "SMO.SweepControl.lvclass">)  [unwired: 5 in]
              n103 = Or(x=w294, y=w295) -> (x .or. y?=w293:bool)
              n104 = while {
                tunnel: w298 -> [w315]
                tunnel: w297 -> [w311]
                tunnel: [w304] -> w292
                tunnel: [w303] -> w291
                tunnel: [w302] -> w290
                i -> [w310]
                stop <- w306 stop-if-true
                w314 = 0  # loop#
                n105 = call "Sweep Control Inner Loop.vi"("error in (no error)"=w315, "inner loop index"=w310, "loop #"=w314, "SweepControl in"=w311) -> ("error out"=w313:errorcluster, "Stop?"=w308:bool, "SweepControl out"=w312:refnum<class "SMO.SweepControl.lvclass">)  [unwired: 5 in]
                n106 = Or(x=w308, y="Stop") -> (x .or. y?=w306:bool)
                n107 = Equal To 0?(x=w310) -> (x = 0?=w309:bool)
                n108 = for {
                  N: "Repeat Experiment" -> [_]
                  tunnel: w313 -> [w324]
                  tunnel: w312 -> [w323]
                  tunnel: w309 -> [w322]
                  tunnel: w306 -> [w320]
                  tunnel: [w318] -> w304
                  tunnel: [w317] -> w303
                  tunnel: [w316] -> w302
                  i -> [w321]
                  stop <- w319 stop-if-true
                  n109 = local read "Stop"() -> (w319:bool)
                  n110 = call "Take Measurement.vi"("stop?"=w320, "initialize?"=w322, "error in (no error)"=w324, "SweepControl in"=w323) -> ("Control Experiment SM"=w316:refnum<class "Control Experiment SM.lvclass">, "Transport out"=w317:refnum<class "SMO.Transport.lvclass">, "SweepControl"=w318:refnum<class "SMO.SweepControl.lvclass">)  [unwired: 4 in, 1 out]
                  "Repeat #" <- w321
                }
              }
            }
          }
        }
        n111 = Bundle By Name(cluster=w258, "Control Experiment"=w257) -> (w261:refnum<class "SMO.SweepControl.lvclass">)
        n112 = Bundle By Name(cluster=w260, "SweepControl"=w261) -> (w259:T18)
        n113 = call <vilib>:"Add State(s) to Queue__jki_lib_state_machine.vi"("State(s) in (\"\")"=w264) -> ("States Out"=w265:string)  [unwired: 14 in]
      }
    }
  }
  "error out" <- w1
